vi "HeaderAction.vi"(0 "InstrClass":refnum<class "ThorCCS200.lvclass"> caption="DNL_LabVIEW Object in", 11 "error in (no error)":errorcluster caption="entrée d'erreur (pas d'erreur)") -> (4 "InstrClassOut":refnum<class "ThorCCS200.lvclass"> caption="DNL_LabVIEW Object out", 6 "DataNames":string[](array[string]), 8 "Instr Name":string, 10 "HeaderString":string, 13 "ArrDisplayNames":string[](array[string]), 14 "DisplayNames":string[](array[string]), 15 "error out":errorcluster caption="sortie d'erreur")   [LabVIEW 2019, in "ThorCCS200.lvclass"]
uses:
  ThorCCS200.lvclass
  C:/Programmes Labview/LabScanV1A/DevicesClass/BaseDevice/BaseDevice.lvclass
  ThorCCS200.lvclass/ThorCCS200.ctl
  BaseDevice/BaseDevice.lvclass
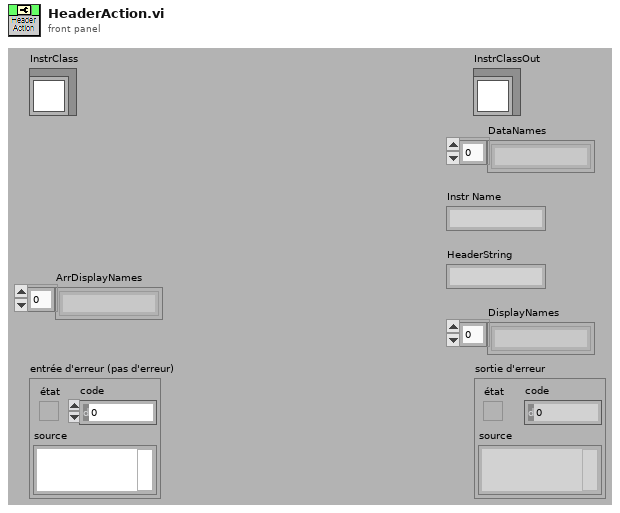
[diagram p1: front panel]
types:
  T1 = typedef "ThorCCS200.lvclass/ThorCCS200_Func.ctl" = enum16{"ReadSpectrum (Acq)"}
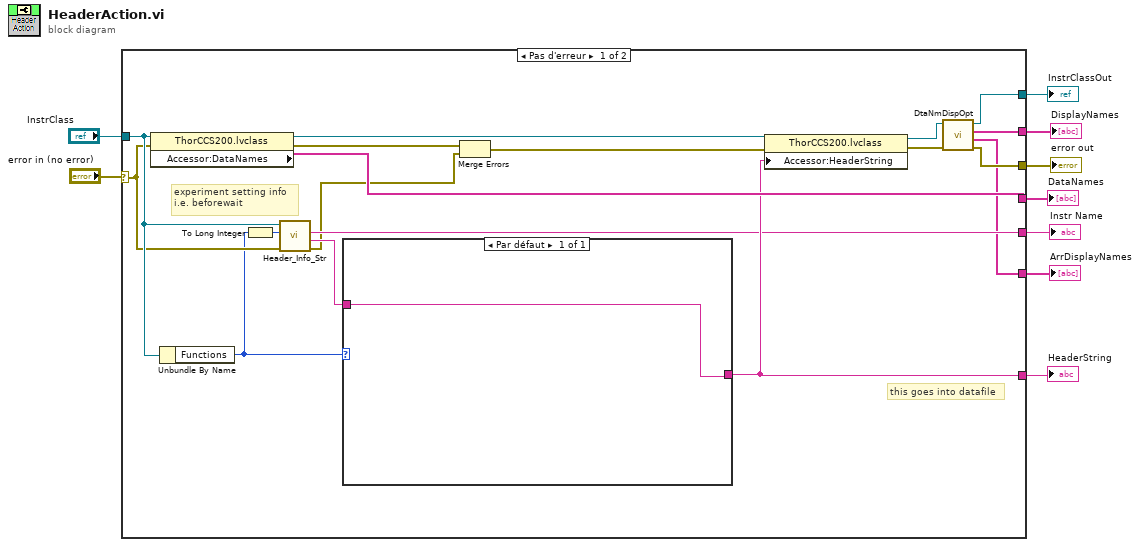
[diagram p0: block diagram]
diagram:
  n1 = case shown="Pas d'erreur" "error in (no error)" {
    selector: "error in (no error)" -> [w15 w29]
    tunnel: [w24 _] -> w8
    tunnel: [w27 _] -> w7
    tunnel: "InstrClass" -> [w18 w30]
    tunnel: [w22 w29] -> w5
    tunnel: [w21 w30] -> w3
    tunnel: [w17 _] -> w4
    tunnel: [w19 _] -> w2
    tunnel: [w10 _] -> w1
    frame No Error {
      # "this goes into datafile"
      # "experiment setting info\ni.e. beforewait"
      n2 = property class="ThorCCS200.lvclass"(reference=w18, error in=w15) -> (reference out=w26:refnum<class "ThorCCS200.lvclass">, error out=w25:errorcluster, "Accessor:DataNames"=w27:string[])
      n3 = Unbundle By Name(w18) -> ("Functions"=w12:T1)
      n4 = To Long Integer(number=w12) -> (32bit integer=w11:i32)
      n5 = call-dynamic "Header_Info_Str.vi"("error in (no error)"=w15, "Functions"=w11, "DefaultDev in"=w18) -> ("error out"=w13:errorcluster, "HdrInfoStr"=w16:string, "InstrumentName"=w17:string)  [unwired: 5 in, 1 out]
      n6 = case shown="Par défaut" w12 {
        tunnel: [w28] -> w24
        tunnel: w16 -> [w28]
        frame Par défaut {
        }
      }
      n7 = Merge Errors(w25, w13) -> (w14:errorcluster)
      n8 = property class="ThorCCS200.lvclass"(reference=w26, error in=w14, "Accessor:HeaderString"=w24) -> (reference out=w20:refnum<class "ThorCCS200.lvclass">, error out=w23:errorcluster)
      n9 = call "DtaNmDispOpt.vi"("error in (no error)"=w23, "BaseDevice en entrée"=w20) -> ("error out"=w22:errorcluster, "ArrDisplayNames"=w10:string[], "DisplayNames"=w19:string[], "BaseDevice en sortie"=w21:refnum<class "ThorCCS200.lvclass">)  [unwired: 6 in]
    }
    frame Error {
    }
  }
  "error out" <- w5
  "InstrClassOut" <- w3
  "DataNames" <- w7
  "HeaderString" <- w8
  "Instr Name" <- w4
  "DisplayNames" <- w2
  "ArrDisplayNames" <- w1
